vi "Auto-Zero.vi"(8 "error in (no error)":errorcluster, 11 "AD4212C in":refnum<class "AD4212C.lvclass">) -> (0 "error out":errorcluster, 3 "AD4212C out":refnum<class "AD4212C.lvclass">)   [LabVIEW 2014, in "AD4212C.lvlib" / "AD4212C.lvclass"]
doc: "Seteo Automático de Auto-Cero para la Balanza."
uses:
  AD4212C.lvclass
  AD4212C.lvclass/AD4212C.ctl
  API/AD4212C Lib.lvlib
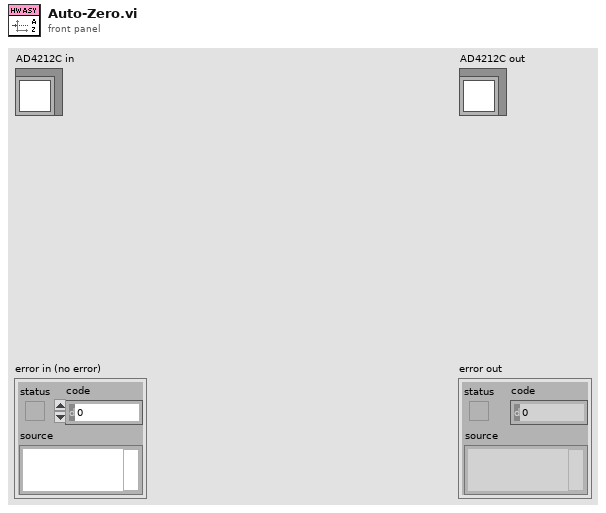
[diagram p1: front panel]
types:
  T1 = typedef "AD4212C Lib.lvlib/Connection Data.ctl" = cluster{"Conection Data":refnum<visa-resource-name>}
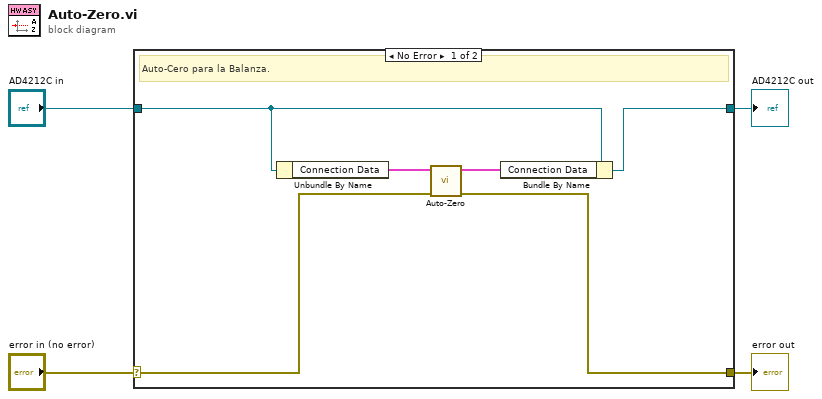
[diagram p0: block diagram]
diagram:
  n1 = case shown="No Error" "error in (no error)" {
    selector: "error in (no error)" -> [w10 w12]
    tunnel: [w9 w12] -> w3
    tunnel: [w5 w11] -> w1
    tunnel: "AD4212C in" -> [w6 w11]
    frame No Error {
      # "Auto-Cero para la Balanza."
      n2 = Unbundle By Name(w6) -> ("Connection Data"=w8:T1)
      n3 = call "Auto-Zero.vi"("error in (no error)"=w10, "VISA resource name In"=w8) -> ("error out"=w9:errorcluster, "VISA resource name Out"=w7:T1)  [unwired: 8 in]
      n4 = Bundle By Name(cluster=w6, "Connection Data"=w7) -> (w5:refnum<class "AD4212C.lvclass">)
    }
    frame Error {
    }
  }
  "error out" <- w3
  "AD4212C out" <- w1
